vi "STD校准信息写入.vi"(8 "Error in":errorcluster caption="Error in (no error)", 10 "校准信息读取":T1 {"校准类型" items=["单点校准"=1, "两点校准"=2, "三点校准"=3]}, 11 "Slave ID":u8=1) -> (0 "error out":errorcluster, 3 "结果字符串":string)   [LabVIEW 2016, in "斯坦道原位多参数.lvlib"]
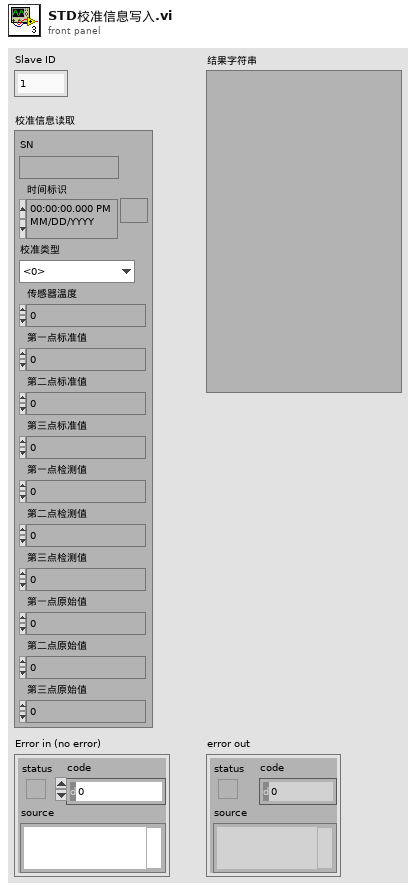
[diagram p1: front panel]
types:
  T1 = cluster{"SN":string, "时间标识":timestamp, "校准类型":u16, "传感器温度":sgl, "第一点标准值":sgl, "第二点标准值":sgl, "第三点标准值":sgl, "第一点检测值":sgl, "第二点检测值":sgl, "第三点检测值":sgl, "第一点原始值":sgl, "第二点原始值":sgl, "第三点原始值":sgl}
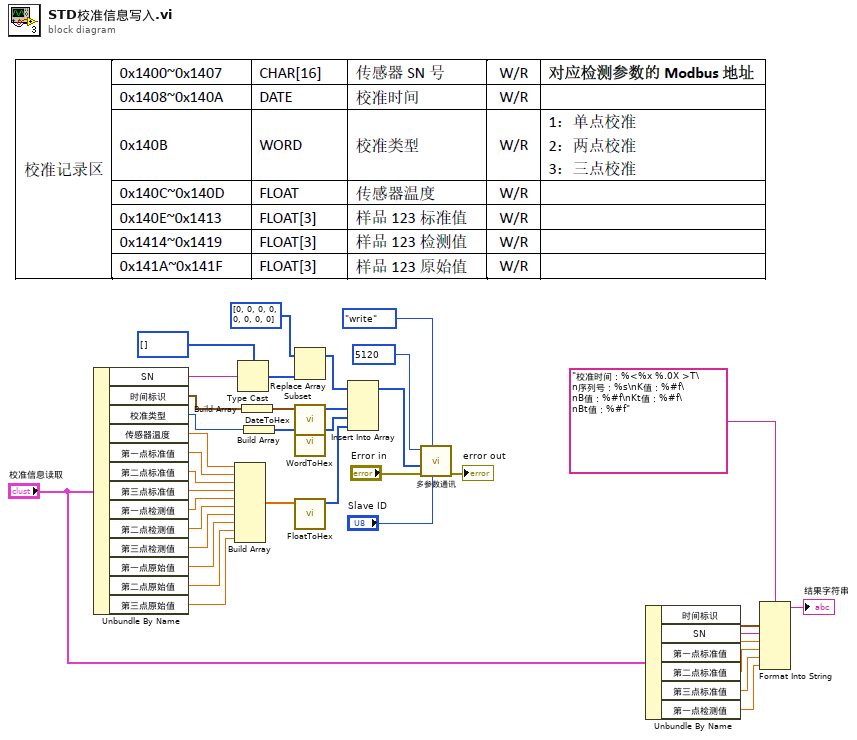
[diagram p0: block diagram]
diagram:
  n1 = Unbundle By Name("校准信息读取") -> ("SN"=w15:string, "时间标识"=w33:timestamp, "校准类型"=w31:u16, "传感器温度"=w29:sgl, "第一点标准值"=w28:sgl, "第二点标准值"=w27:sgl, "第三点标准值"=w26:sgl, "第一点检测值"=w25:sgl, "第二点检测值"=w24:sgl, "第三点检测值"=w23:sgl, "第一点原始值"=w22:sgl, "第二点原始值"=w21:sgl, "第三点原始值"=w20:sgl)
  n2 = Build Array(w29, w28, w27, w26, w25, w24, w23, w22, w21, w20) -> (w19:sgl[])
  n3 = Type Cast(type=u16[] [], x=w15) -> (*(type *) &x=w11:u16[])
  n4 = Build Array(w33) -> (w32:timestamp[])
  n5 = Build Array(w31) -> (w30:u16[])
  n6 = Replace Array Subset(array=u16[] [0, 0, 0, 0, 0, 0, 0, 0], new element=w11) -> (w10:u16[])  [unwired: 1 in]
  n7 = call "DateToHex.vi"("DATE"=w32) -> ("数组"=w13:u16[])  [unwired: 10 in]
  n8 = call "WordToHex.vi"("WORD"=w30) -> ("数组"=w18:u16[])  [unwired: 10 in]
  n9 = call "FloatToHex.vi"("浮点数"=w19) -> ("DCBA整形输出"=w17:u16[])  [unwired: 10 in]
  n10 = Insert Into Array(array=w10, new element #1=w13, new element #2=w18, new element #3=w17) -> (w16:u16[])  [unwired: 1 in]
  n11 = call "多参数通讯.vi"("Slave ID"="Slave ID", "STEP"=enum16{"open", "read", "write", "close"}."write", "Error in"="Error in", "values"=w16, "starting address"=u16 5120) -> ("error out"=→"error out":errorcluster)  [unwired: 4 in, 2 out]
  n12 = Unbundle By Name("校准信息读取") -> ("时间标识"=w8:timestamp, "SN"=w7:string, "第一点标准值"=w6:sgl, "第二点标准值"=w5:sgl, "第三点标准值"=w4:sgl, "第一点检测值"=w3:sgl)
  n13 = Format Into String(format string="校准时间：%<%x %.0X >T\n序列号：%s\nK值：%#f\nB值：%#f\nKt值：%#f\nBt值：%#f" ("格式字符串"), w8, w7, w6, w5, w4, w3) -> (resulting string=→"结果字符串":string)  [unwired: 2 in, 1 out]
